vi "Insert Into Array.vi"() -> ()   [LabVIEW 2017]
panel:
  out "output array":dbl[](array[numeric])
  in  "index":i32
  in  "array":dbl[](array[numeric])
  # "Insert into Array"
  # "Works very similar to \nReplace Array Subset,\nexcept instead of replacing the\nelement, it adds it instead at the index point."
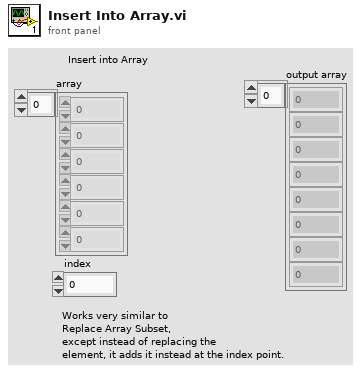
[diagram p1: front panel]
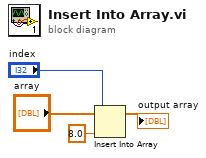
[diagram p0: block diagram]
diagram:
  n1 = Insert Into Array(array="array", index="index", new element=8.0 ("new element/subarray")) -> (→"output array":dbl[])
